vi "Pre-append object type byte.vi"(10 "data in":u8[](array[numeric]), 11 "Format byte":T1 items=["nil"=192, "UINT8"=204, "UINT16"=205, "UINT32"=206, "UINT64"=207, "INT8"=208, "INT16"=209, "INT32"=210, "INT64"=211]) -> (3 "bytes add":u8[](array[numeric]) format="%x")   [LabVIEW 2020, in "wamplv.lvlib" / "MessagePack.lvclass"]
uses:
  MessagePack.lvclass
  Format bytes.ctl
  MessagePack.lvclass/MessagePack.ctl
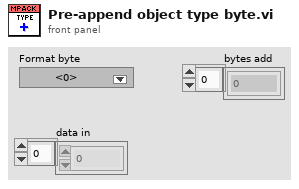
[diagram p1: front panel]
types:
  T1 = typedef "wamplv.lvlib/MessagePack.lvclass/Format bytes.ctl" = u8
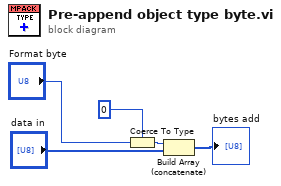
[diagram p0: block diagram]
diagram:
  n1 = Coerce To Type(0:"Format byte", 1:u8 0) -> (2:w2:u8)
  n2 = Build Array (concatenate)(w2, "data in") -> (→"bytes add":u8[])
